vi "LINX - Analog Read 1 Channel (TCP).vi"() -> ()   [LabVIEW 2020]
doc: "Manually blink and LED attached to a digital output channel of a LINX device by clicking and LED control in LabVIEW."
uses:
  <vilib>/MakerHub/LINX/Private/Device/Type Defs/TCP Config.ctl
  <vilib>/MakerHub/LINX/Public/Peripherals/Analog/Analog Read 1 Chan.vi
  <vilib>/MakerHub/LINX/Public/Peripherals/Analog/Analog Read N Chans.vi
  <vilib>/MakerHub/LINX/Private/Local IO/LinxAnalogRead.vi
  <vilib>/MakerHub/LINX/Public/Utilities/Check Channel.vi
  <vilib>/MakerHub/LINX/Public/Utilities/Open TCP.vi
  <vilib>/MakerHub/LINX/Private/Utilties/Generate Error.vi
  <vilib>/MakerHub/LINX/LMH-LINX.lvlib
  <vilib>/MakerHub/LINX/Private/Device/Device.lvlib
panel:
  out "Analog Data":dbl(graph)
  out "Loop Rate (Hz)":u32
  in  "TCP Configuration":T1
  in  "GPIO":u8=13
  in  "Stop Button":bool
  # "LINX Device Settings"
  # "Analog Read 1 Channel Example (TCP)\n\nThis is a sample of graph display of the analog input connected to GPIO.\n\nInstructions\n1. Select the TCP Configuration associated with the LINX Device.\n2. Select the GPIO connected to Analog Input.\n3. Click the Run Arrow."
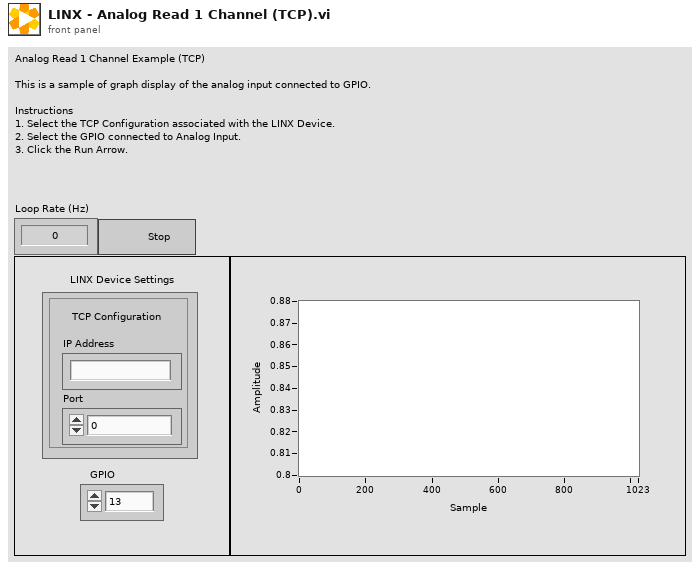
[diagram p1: front panel]
types:
  T1 = typedef "LMH-LINX.lvlib/Device.lvlib/TCP Config.ctl" = cluster{"IP Address":string, "Port":u16}
  T2 = typedef "LMH-LINX.lvlib/LINX Ref.ctl" = cluster{"IO":T3, "Interface":T4, "LINX Device Config":T5}
  T3 = typedef "LMH-LINX.lvlib/Platform.ctl" = enum16{"Remote", "Local"}
  T4 = typedef "LMH-LINX.lvlib/Interface.ctl" = enum16{"Serial", "TCP"}
  T5 = typedef "LMH-LINX.lvlib/Device.lvlib/LINX Device Config.ctl" = cluster{"Interface":T4, "COM Port":refnum<visa-resource-name>, "TCP Configuration":T1, "Device Family":u8, "Device ID":u8, "Device Name":string, "TCP Ref":refnum<k5>, "Channels":T6}
  T6 = typedef "LMH-LINX.lvlib/Channels.ctl" = cluster{"DI":u8[], "DO":u8[], "AI":u8[], "AO":u8[], "PWM":u8[], "QE":u8[], "UART":u8[], "I2C 2":u8[], "SPI":u8[], "CAN":u8[], "Servo":u8[], "AI Ref (V)":dbl, "AI Resolution (Bits)":u8, "AO Ref (V)":dbl, "AO Resolution (Bits)":u8}
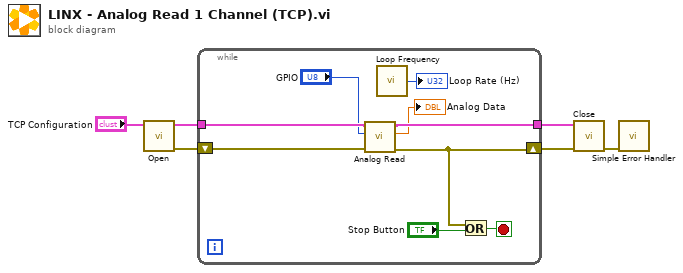
[diagram p0: block diagram]
diagram:
  n1 = call-poly <vilib>:"Open.vi"("TCP Configuration"="TCP Configuration") -> ("Error Out"=w5:errorcluster, "LINX Resource"=w6:T2)  [unwired: 8 in, 1 out]
  n2 = while {
    tunnel: w6 -> [w13]
    tunnel: [w12] -> w4
    shift-right: [w10] -> w3
    shift-left: w5 -> [w11]
    stop <- w15 stop-if-true
    n3 = call-poly <vilib>:"Analog Read.vi"("Error In"=w11, "Analog Channel"="GPIO", "LINX Resource"=w13) -> ("Error Out"=w10:errorcluster, "Voltage"=→"Analog Data":dbl, "LINX Resource"=w12:T2)  [unwired: 5 in, 1 out]
    n4 = call <vilib>:"Loop Frequency.vi"() -> ("Loop Rate (Hz)"=→"Loop Rate (Hz)":u32)
    n5 = Or(x=w10, y="Stop Button") -> (x .or. y?=w15:bool)
  }
  n6 = call <vilib>:"Close.vi"("Error In"=w3, "LINX Resource"=w4) -> ("Error Out"=w2:errorcluster)  [unwired: 9 in]
  n7 = call <vilib>:"Simple Error Handler.vi"("error in (no error)"=w2) -> ()  [unwired: 4 in, 5 out]
